vi "Calculate Percentage.vi"(11 "1DArray":bool[](array[boolean])) -> (3 "Percentage":dbl)   [LabVIEW 2021, in "Bananas.lvlib" / "Pips.lvclass"]
uses:
  Pips.lvclass
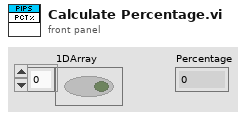
[diagram p1: front panel]
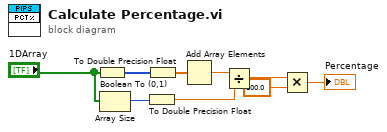
[diagram p0: block diagram]
diagram:
  n1 = Boolean To (0,1)(Boolean="1DArray") -> (0, 1=w2:i16[])
  n2 = Array Size(array="1DArray") -> (size(s)=w1:i32)
  n3 = To Double Precision Float(number=w1) -> (double precision float=w8:dbl)
  n4 = To Double Precision Float(number=w2) -> (double precision float=w4:dbl[])
  n5 = Add Array Elements(numeric array=w4) -> (sum=w3:dbl)
  n6 = Divide(x=w3, y=w8) -> (x/y=w5:dbl)
  n7 = Multiply(x=w5, y=100.0) -> (x*y=→"Percentage":dbl)
